vi "G#MethodTemplates_GetClassAttributesToModify.vi"(0 "reference in":refnum<class "G#BaseTemplateG3.lvclass">, 3 "timeout in ms (-1)":i32=-1, 5 "error in (no error)":errorcluster) -> (14 "reference out":refnum<class "G#BaseTemplateG3.lvclass">, 15 "class attributes ref":T2, 16 "class attributes":T1, 17 "timeout":bool, 18 "created new":bool, 19 "error out":errorcluster)   [LabVIEW 2020, in "G#MethodTemplates.lvclass"]
doc: "This VI returns the attributes associated with this class or subclass object reference and places a lock on the object.\n\nIf the object is currently locked for modification by another method, 'Timeout' specifies how long the VI should wait to receive access to the object. The default value waits until the object becomes available.\n\nYou must use this class SetModifiedAttributes VI to set the object's data and release the lock."
uses:
  G#MethodTemplates.lvclass
  G#BaseTemplateG3/G#BaseTemplateG3.lvclass
  ClassAttributesRef.ctl
  protected/ClassAttributes.ctl
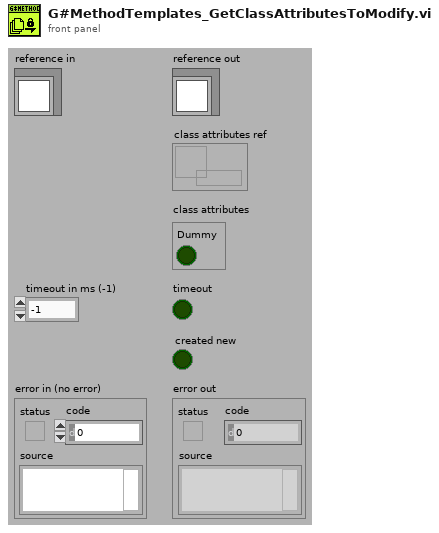
[diagram p1: front panel]
types:
  T1 = typedef "G#MethodTemplates.lvclass/ClassAttributes.ctl" = cluster{"Dummy":bool}
  T2 = typedef "G#MethodTemplates.lvclass/ClassAttributesRef.ctl" = refnum<data-value>
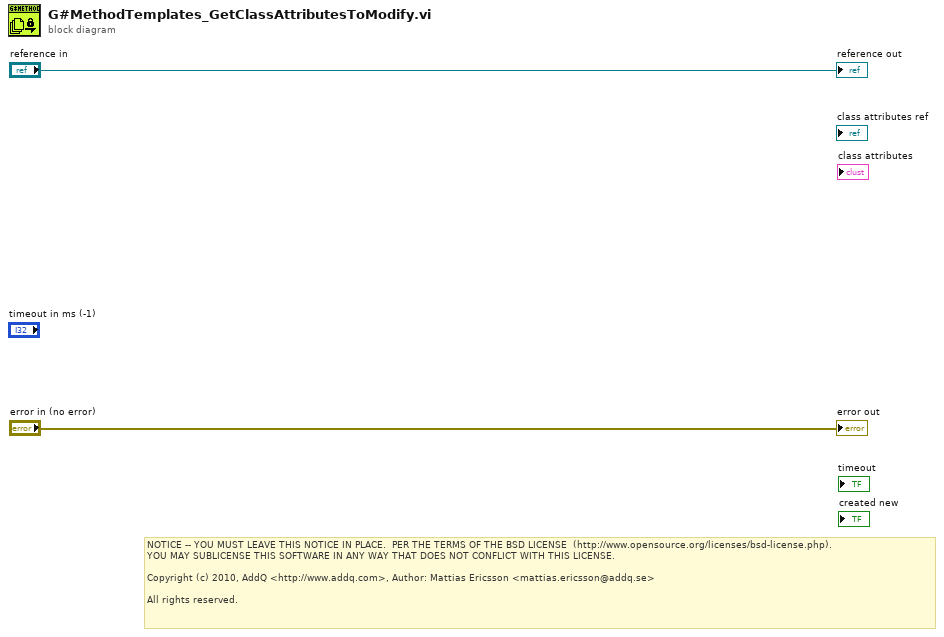
[diagram p0: block diagram]
diagram:
  # "NOTICE -- YOU MUST LEAVE THIS NOTICE IN PLACE.  PER THE TERMS OF THE BSD LICENSE  (http://www.opensource.org/licenses/bsd-license.php).\nYOU MAY SUBLICENSE THIS SOFTWARE IN ANY WAY THAT DOES NOT CONFLICT WITH THIS LICENSE.\n\nCopyright (c) 2010, AddQ <http://www.addq.com>, Author: Mattias Ericsson <mattias.ericsson@addq.se>\n\nAll rights reserved."
  "error out" <- "error in (no error)"
  "reference out" <- "reference in"
